vi "Start TLS.vi"(6 "server certificate validation":enum32{"Any Trusted CA", "None"}(ring), 7 "timeout ms":i32, 8 "error in (no error)":errorcluster, 9 "server hostname":string, 10 "immutable TLS configuration":refnum<k36>, 11 "TCP Stream in":refnum<class "TCP Stream.lvclass">) -> (0 "error out":errorcluster, 2 "server certificate chain":cluster{"certificate":u8[]}[](array[cluster]), 3 "TCP Stream out":refnum<class "TCP Stream.lvclass">)   [LabVIEW 2020, in "Stream-TCP.lvlib" / "TCP Stream.lvclass"]
uses:
  TCP Stream.lvclass
  TCP Stream.lvclass/TCP Stream.ctl
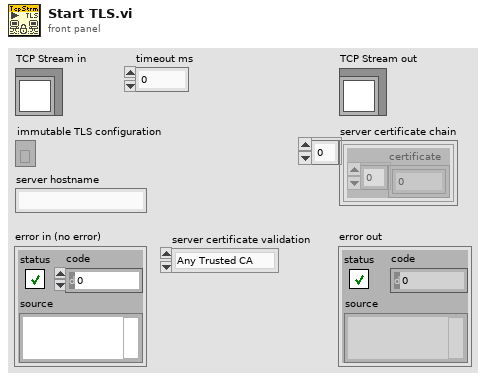
[diagram p1: front panel]
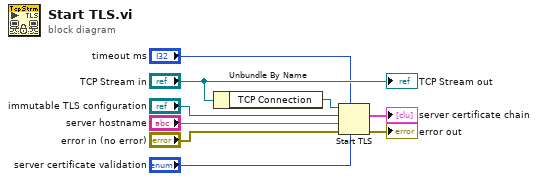
[diagram p0: block diagram]
diagram:
  n1 = Unbundle By Name("TCP Stream in") -> ("TCP Connection"=w3:refnum<k5>)
  n2 = Start TLS(6:"server certificate validation", 7:"timeout ms", 8:"error in (no error)", 9:"server hostname", 10:"immutable TLS configuration", 11:w3) -> (0:→"error out":errorcluster, 2:→"server certificate chain":cluster{"certificate":u8[]}[])  [unwired: 1 out]
  "TCP Stream out" <- "TCP Stream in"
